vi "pushme.vi"() -> ()   [LabVIEW 2013]
panel:
  in  "Color Box":u32(colorbox)
  in  "stop 2":bool
  out "Waveform Chart":dbl(graph)
  in  "stop":bool
  in  "Blinking":bool
  in  "OK Button":bool
  in  "Visible":bool
  in  "Push Me":bool
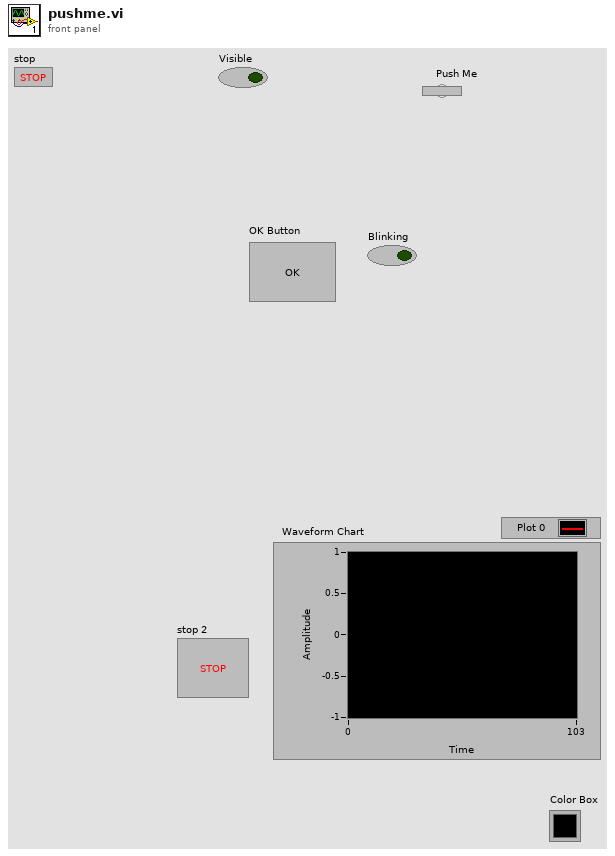
[diagram p1: front panel]
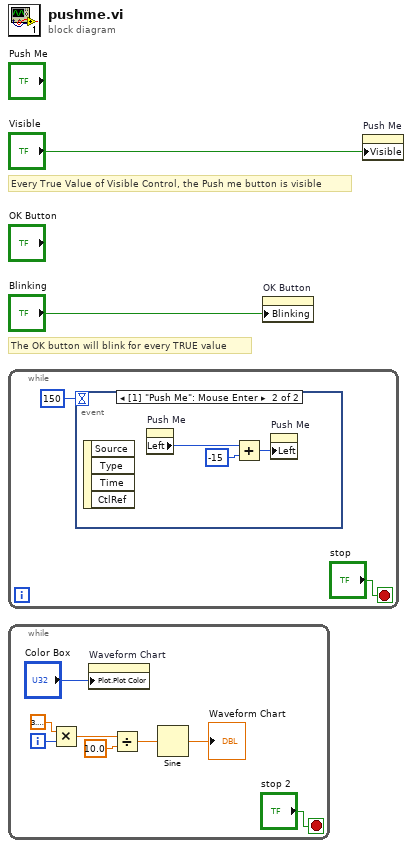
[diagram p0: block diagram]
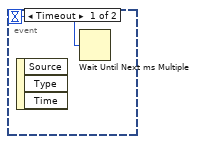
[diagram p2: hidden frame]
diagram:
  # "The OK button will blink for every TRUE value"
  # "Every True Value of Visible Control, the Push me button is visible"
  n1 = while {
    stop <- "stop" stop-if-true
    n2 = event shown="[1] \"Push Me\": Mouse Enter" {
      selector: _ -> [_ _]
      dyn-events: _ -> [_ _]
      timeout: u32 150 ("millisecond multiple") -> [w5 _]
      event Timeout {
        n3 = event-data() -> ()  [unwired: 1 in, 3 out]
        n4 = Wait Until Next ms Multiple(millisecond multiple=w5) -> ()  [unwired: 1 out]
      }
      event "Push Me": Mouse Enter {
        n5 = event-data() -> ()  [unwired: 1 in, 4 out]
        n6 = property on="Push Me" class="Bool (strict)"() -> ("Left"=w8:i32)  [unwired: 2 in, 2 out]
        n7 = Add(x=w8, y=-15) -> (x+y=w6:i32)
        n8 = property on="Push Me" class="Bool (strict)"("Left"=w6) -> ()  [unwired: 2 in, 2 out]
      }
    }
  }
  n9 = while {
    i -> [w12]
    stop <- "stop 2" stop-if-true
    n10 = Multiply(x=3.141592653589793, y=w12) -> (x*y=w11:dbl)
    n11 = property on="Waveform Chart" class="WFChart (strict)"("Plot.Plot Color"="Color Box") -> ()  [unwired: 2 in, 2 out]
    n12 = Divide(x=w11, y=10.0) -> (x/y=w9:dbl)
    n13 = Sine(x=w9) -> (sin(x)=→"Waveform Chart":dbl)
  }
  n14 = property on="OK Button" class="Bool"("Blinking"="Blinking") -> ()  [unwired: 2 in, 2 out]
  n15 = property on="Push Me" class="Bool (strict)"("Visible"="Visible") -> ()  [unwired: 2 in, 2 out]
